vi "HWTestMain.vi"() -> ()   [LabVIEW 2015]
uses:
  <vilib>/DAQmx/write.llb/DAQmx Write (Analog DBL 1Chan 1Samp).vi
  <vilib>/DAQmx/read.llb/DAQmx Read (Analog 1D Wfm NChan NSamp).vi
  <vilib>/Analysis/baseanly.llb/Mean (DBL).vi
  <vilib>/DAQmx/create/channels.llb/DAQmx Create Channel (AI-Voltage-Basic).vi
  <vilib>/DAQmx/configure/timing.llb/DAQmx Timing (Sample Clock).vi
  <vilib>/DAQmx/create/channels.llb/DAQmx Create Channel (AO-Voltage-Basic).vi
  <vilib>/DAQmx/miscellaneous.llb/DAQmx Fill In Error Info.vi
  <vilib>/Analysis/2dsp.llb/Decimate (continuous, DBL).vi
  <resource>/objmgr/daqmx.rc
  <vilib>/Analysis/NI_AALBase.lvlib
  <vilib>/Analysis/NI_AALPro.lvlib
panel:
  out "PPG":dbl[](graph) caption="Filtered_HS"
  out "RawDisp_HSR":dbl[](graph) caption="Filtered_TA"
  out "RawDisp_QCR":dbl[](graph) caption="Filtered_GL"
  out "RawDisp_HSL":dbl[](graph) caption="Filtered_QC"
  out "RawDisp_QCL":dbl[](graph) caption="Filtered_HS"
  # "HS Right"
  # "QC Right"
  # "QC Left"
  # "HS Left"
  # "PPG Raw"
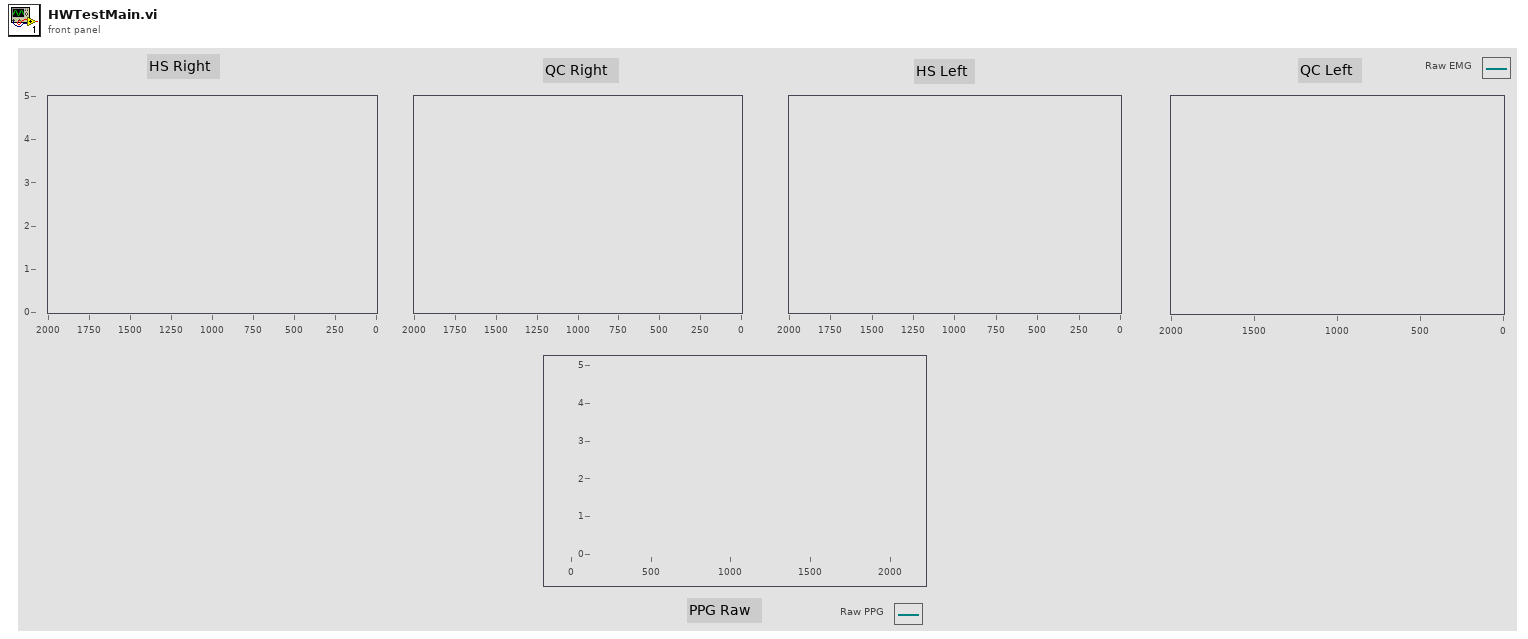
[diagram p1: front panel]
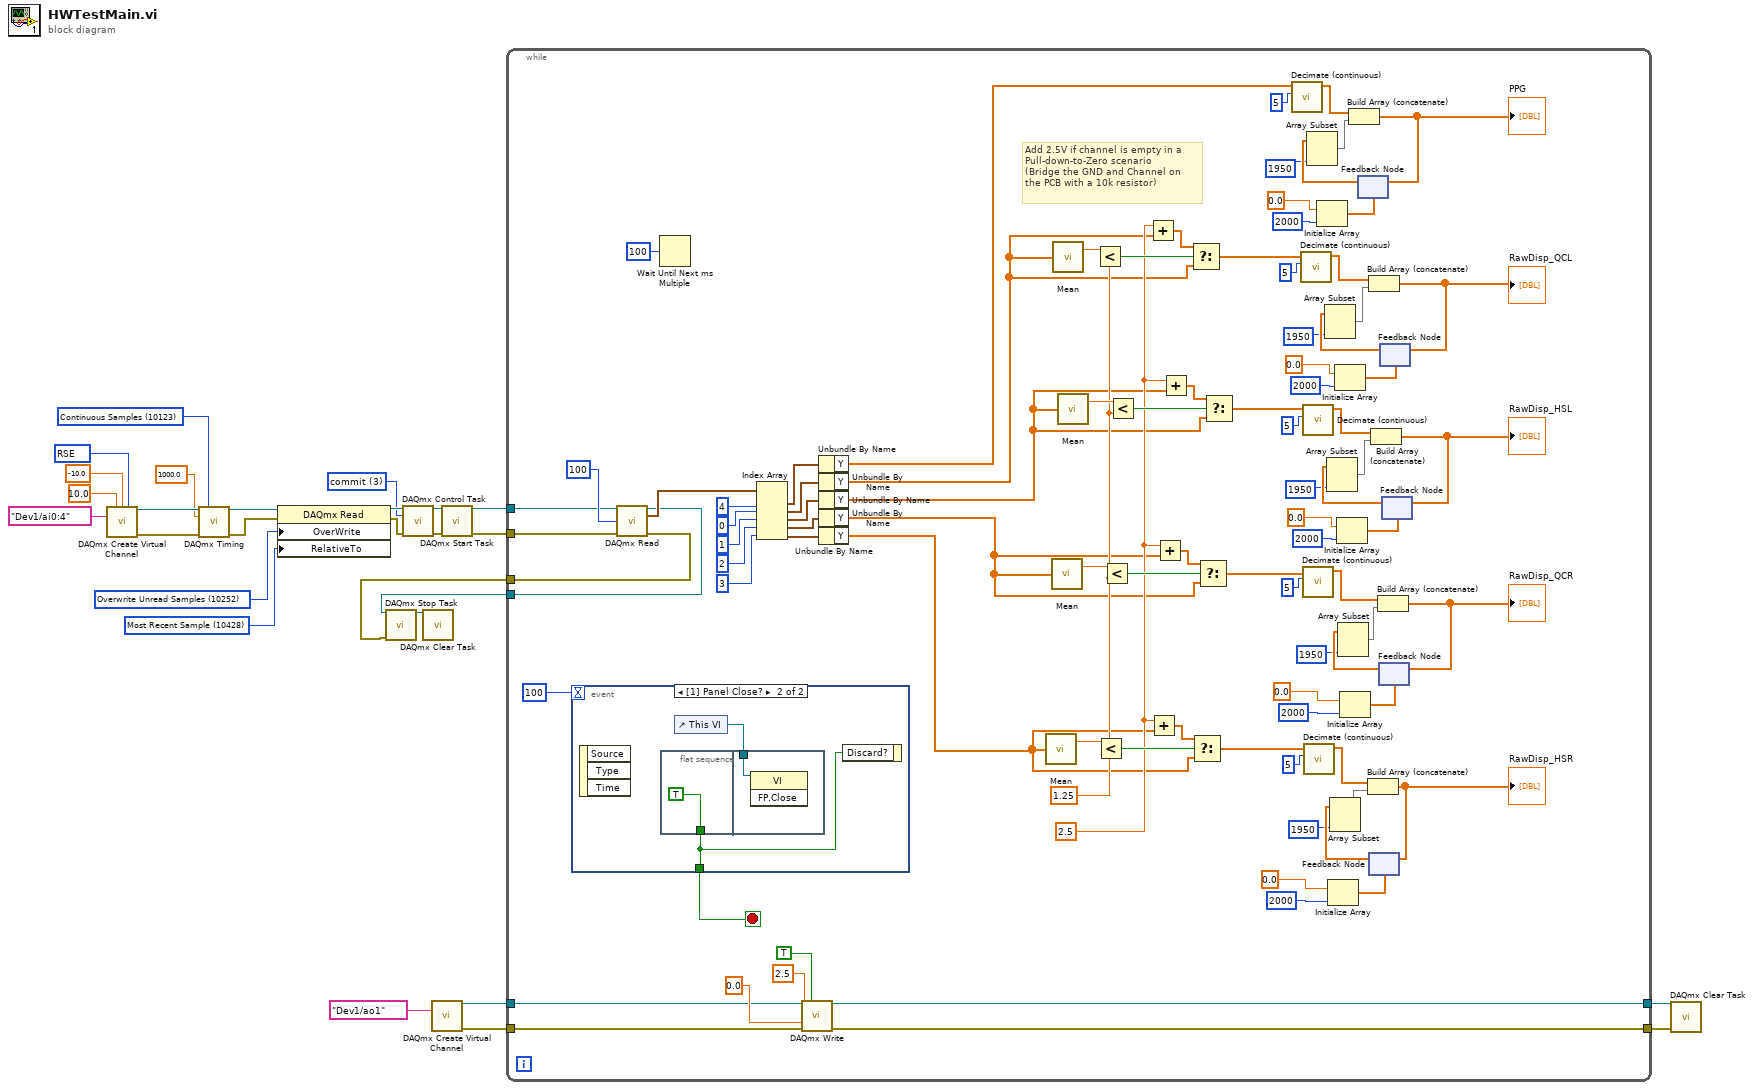
[diagram p0: block diagram]
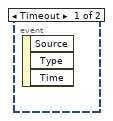
[diagram p2: hidden frame]
diagram:
  w10 = 3 items=["verify"=2, "reserve"=4, "commit"=3, "unreserve"=5, "abort"=6] ("action")
  w21 = 10083 items=["Default"=-1, "RSE"=10083, "NRSE"=10078, "Differential"=10106, "Pseudodifferential"=12529] ("input terminal configuration")
  w16 = 10428 items=["First Sample"=10424, "Current Read Position"=10425, "Reference Trigger"=10426, "First Pretrigger Sample"=10427, "Most Recent Sample"=10428] ("RelativeTo")
  w17 = 10252 items=["Overwrite Unread Samples"=10252, "Do Not Overwrite Unread Samples"=10159] ("OverWrite")
  w22 = 10123 items=["Finite Samples"=10178, "Continuous Samples"=10123, "Hardware Timed Single Point"=12522] ("sample mode")
  n1 = call-poly <vilib>:"DAQmx Create Virtual Channel.vi"("maximum value"=10.0, "minimum value"=-10.0, "input terminal configuration"=w21, "physical channels"=tag "Dev1/ai0:4") -> ("task out"=w27:refnum<k21>, "error out"=w26:errorcluster)  [unwired: 10 in]
  n2 = call-poly <vilib>:"DAQmx Timing.vi"("task/channels in"=w27, "sample mode"=w22, "rate"=1000.0, "error in"=w26) -> ("task out"=w19:refnum<k21>, "error out"=w18:errorcluster)  [unwired: 10 in]
  n3 = property class="DAQmx Read"(reference=w19, error in=w18, "OverWrite"=w17, "RelativeTo"=w16) -> (reference out=w12:refnum<k21>, error out=w11:errorcluster)
  n4 = call <vilib>:"DAQmx Control Task.vi"("task/channels in"=w12, "action"=w10, "error in"=w11) -> ("task out"=w14:refnum<k21>, "error out"=w13:errorcluster)  [unwired: 11 in]
  n5 = call-poly <vilib>:"DAQmx Create Virtual Channel.vi"("physical channels"=tag "Dev1/ao1") -> ("task out"=w2:refnum<k21>, "error out"=w1:errorcluster)  [unwired: 13 in]
  n6 = call <vilib>:"DAQmx Start Task.vi"("task/channels in"=w14, "error in"=w13) -> ("task out"=w9:refnum<k21>, "error out"=w8:errorcluster)  [unwired: 12 in]
  n7 = while {
    tunnel: w9 -> [w110]
    tunnel: w8 -> [w109]
    tunnel: [w108] -> w7
    tunnel: [w107] -> w6
    tunnel: [w32] -> w4
    tunnel: [w31] -> w3
    tunnel: w2 -> [w30]
    tunnel: w1 -> [w29]
    stop <- w121 stop-if-true
    w92 = 1.25 ("x")
    w93 = 2.5 ("x")
    # "Add 2.5V if channel is empty in a \nPull-down-to-Zero scenario\n(Bridge the GND and Channel on \nthe PCB with a 10k resistor)"
    n8 = event shown="[1] Panel Close?" {
      selector: _ -> [_ _]
      dyn-events: _ -> [_ _]
      timeout: 100 -> [_ _]
      tunnel: [_ w123] -> w121
      event Timeout {
        n9 = event-data() -> ()  [unwired: 1 in, 3 out]
      }
      event Panel Close? {
        n10 = event-data() -> ()  [unwired: 1 in, 3 out]
        n11 = flat-sequence {
          tunnel: [TRUE] -> w123
          tunnel: w122 -> [w125]
          frame #0 {
          }
          frame #1 {
            n12 = invoke class="VI" method="FP.Close"(reference=w125) -> ()  [unwired: 2 in, 3 out]
          }
        }
        n13 = control-ref of="This VI"() -> (w122:refnum<vi>)
        n14 = event-data("Discard?"=w123) -> ()  [unwired: 1 in, 1 out]
      }
    }
    n15 = call-poly <vilib>:"DAQmx Read.vi"("task/channels in"=w110, "number of samples per channel"=100, "error in"=w109) -> ("task out"=w107:refnum<k21>, "data"=w115:waveform(dbl)[], "error out"=w108:errorcluster)  [unwired: 10 in]
    n16 = Wait Until Next ms Multiple(millisecond multiple=u32 100) -> ()  [unwired: 1 out]
    n17 = Index Array(array=w115, index #1=4 ("index"), index #2=0 ("index"), index #3=1 ("index"), index #4=2 ("index"), index #5=3 ("index")) -> (element #1=w119:waveform(dbl), element #2=w118:waveform(dbl), element #3=w116:waveform(dbl), element #4=w117:waveform(dbl), element #5=w106:waveform(dbl))
    n18 = call-poly <vilib>:"DAQmx Write.vi"("task/channels in"=w30, "auto start"=TRUE, "data"=2.5, "timeout"=0.0, "error in"=w29) -> ("task out"=w32:refnum<k21>, "error out"=w31:errorcluster)  [unwired: 8 in, 1 out]
    n19 = Unbundle By Name(w119) -> ("Y"=w80:dbl[])
    n20 = Unbundle By Name(w118) -> ("Y"=w70:dbl[])
    n21 = Unbundle By Name(w116) -> ("Y"=w89:dbl[])
    n22 = Unbundle By Name(w117) -> ("Y"=w90:dbl[])
    n23 = Unbundle By Name(w106) -> ("Y"=w91:dbl[])
    n24 = call-poly <vilib>:"Mean.vi"("X"=w91) -> ("mean"=w100:dbl)  [unwired: 1 out]
    n25 = call-poly <vilib>:"Mean.vi"("X"=w90) -> ("mean"=w103:dbl)  [unwired: 1 out]
    n26 = call-poly <vilib>:"Mean.vi"("X"=w70) -> ("mean"=w94:dbl)  [unwired: 1 out]
    n27 = call-poly <vilib>:"Mean.vi"("X"=w89) -> ("mean"=w97:dbl)  [unwired: 1 out]
    n28 = Less?(x=w94, y=w92) -> (x < y?=w95:bool)
    n29 = Less?(x=w100, y=w92) -> (x < y?=w101:bool)
    n30 = Less?(x=w103, y=w92) -> (x < y?=w104:bool)
    n31 = Less?(x=w97, y=w92) -> (x < y?=w98:bool)
    n32 = Add(x=w93, y=w70) -> (x+y=w96:dbl[])
    n33 = Add(x=w93, y=w91) -> (x+y=w102:dbl[])
    n34 = Add(x=w93, y=w90) -> (x+y=w105:dbl[])
    n35 = Add(x=w93, y=w89) -> (x+y=w99:dbl[])
    n36 = Select(t=w96, s=w95, f=w70) -> (s? t:f=w71:dbl[])
    n37 = Select(t=w102, s=w101, f=w91) -> (s? t:f=w43:dbl[])
    n38 = Select(t=w105, s=w104, f=w90) -> (s? t:f=w52:dbl[])
    n39 = Select(t=w99, s=w98, f=w89) -> (s? t:f=w61:dbl[])
    n40 = call-poly <vilib>:"Decimate (continuous).vi"("decimating factor"=5, "X"=w80) -> ("Decimated Array"=w82:dbl[])  [unwired: 8 in, 1 out]
    n41 = call-poly <vilib>:"Decimate (continuous).vi"("decimating factor"=5, "X"=w71) -> ("Decimated Array"=w73:dbl[])  [unwired: 8 in, 1 out]
    n42 = call-poly <vilib>:"Decimate (continuous).vi"("decimating factor"=5, "X"=w61) -> ("Decimated Array"=w63:dbl[])  [unwired: 8 in, 1 out]
    n43 = call-poly <vilib>:"Decimate (continuous).vi"("decimating factor"=5, "X"=w52) -> ("Decimated Array"=w54:dbl[])  [unwired: 8 in, 1 out]
    n44 = call-poly <vilib>:"Decimate (continuous).vi"("decimating factor"=5, "X"=w43) -> ("Decimated Array"=w45:dbl[])  [unwired: 8 in, 1 out]
    n45 = Initialize Array(0.0 ("element"), 2000 ("dimension size")) -> (w88:dbl[])
    n46 = Initialize Array(0.0 ("element"), 2000 ("dimension size")) -> (w51:dbl[])
    n47 = Initialize Array(0.0 ("element"), 2000 ("dimension size")) -> (w79:dbl[])
    n48 = Initialize Array(0.0 ("element"), 2000 ("dimension size")) -> (w69:dbl[])
    n49 = Initialize Array(0.0 ("element"), 2000 ("dimension size")) -> (w60:dbl[])
    n50 = feedback #1(w88) -> (w85:dbl[])
    n51 = Array Subset(array=w85, length=1950 ("index")) -> (w83:dbl[])  [unwired: 1 in]
    n52 = Build Array (concatenate)(w82, w83) -> (w42:dbl[])
    "PPG" <- w42
    n53 = feedback-in #1(w42) -> ()
    n54 = feedback #2(w51) -> (w48:dbl[])
    n55 = Array Subset(array=w48, length=1950 ("index")) -> (w46:dbl[])  [unwired: 1 in]
    n56 = Build Array (concatenate)(w45, w46) -> (w38:dbl[])
    "RawDisp_HSR" <- w38
    n57 = feedback-in #2(w38) -> ()
    n58 = feedback #3(w60) -> (w57:dbl[])
    n59 = Array Subset(array=w57, length=1950 ("index")) -> (w55:dbl[])  [unwired: 1 in]
    n60 = Build Array (concatenate)(w54, w55) -> (w39:dbl[])
    "RawDisp_QCR" <- w39
    n61 = feedback-in #3(w39) -> ()
    n62 = feedback #4(w79) -> (w76:dbl[])
    n63 = Array Subset(array=w76, length=1950 ("index")) -> (w74:dbl[])  [unwired: 1 in]
    n64 = Build Array (concatenate)(w73, w74) -> (w41:dbl[])
    "RawDisp_QCL" <- w41
    n65 = feedback-in #4(w41) -> ()
    n66 = feedback #5(w69) -> (w66:dbl[])
    n67 = Array Subset(array=w66, length=1950 ("index")) -> (w64:dbl[])  [unwired: 1 in]
    n68 = Build Array (concatenate)(w63, w64) -> (w40:dbl[])
    "RawDisp_HSL" <- w40
    n69 = feedback-in #5(w40) -> ()
  }
  n70 = call <vilib>:"DAQmx Stop Task.vi"("task/channels in"=w6, "error in"=w7) -> ("task out"=w15:refnum<k21>)  [unwired: 12 in, 1 out]
  n71 = call <vilib>:"DAQmx Clear Task.vi"("task in"=w15) -> ()  [unwired: 14 in, 1 out]
  n72 = call <vilib>:"DAQmx Clear Task.vi"("task in"=w4, "error in"=w3) -> ()  [unwired: 13 in, 1 out]
